vi "main_vi.vi"() -> ()   [LabVIEW 2015]
uses:
  <vilib>/Enthought/Python Integration Toolkit/api/Console Visibility.ctl
  <vilib>/Enthought/Python Integration Toolkit/api/Unpack Double.vi
  <vilib>/Enthought/Python Integration Toolkit/Python Integration Toolkit.lvlib
panel:
  out "State":string
  out "Value":dbl
  in  "Console Visibility":T1=enum."Hide Console"
  in  "Path to Python Module (.py File)":path=path ""
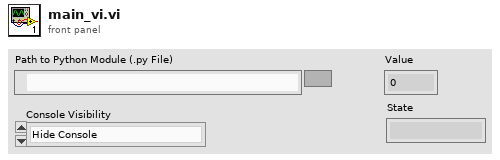
[diagram p1: front panel]
types:
  T1 = typedef "Python Integration Toolkit.lvlib/Console Visibility.ctl" = enum16{"Show Console", "Show Console While Running", "Hide Console"}
  T2 = typedef "Python Integration Toolkit.lvlib/Session ID.ctl" = u64
  T3 = typedef "Python Integration Toolkit.lvlib/Python Objects.ctl" = variant
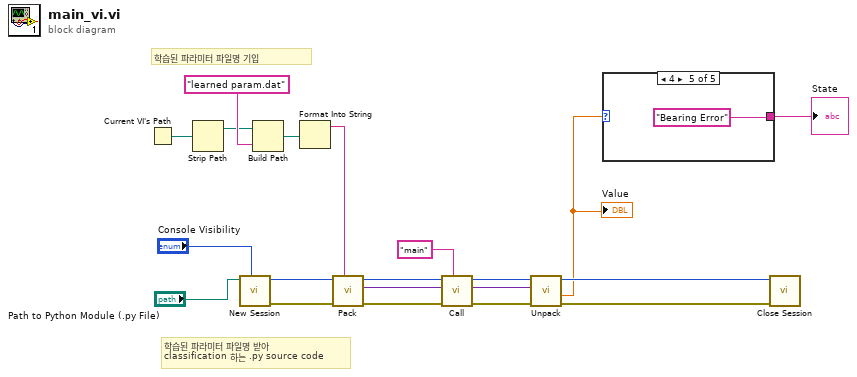
[diagram p0: block diagram]
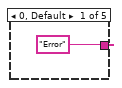
[diagram p2: hidden frame]
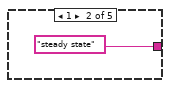
[diagram p3: hidden frame]
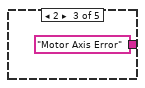
[diagram p4: hidden frame]
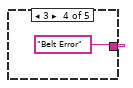
[diagram p5: hidden frame]
diagram:
  # "학습된 파라미터 파일명 받아 \nclassification 하는 .py source code"
  # "학습된 파라미터 파일명 기입"
  n1 = Current VI's Path() -> (path=w14:path)
  n2 = Strip Path(path=w14) -> (stripped path=w12:path)  [unwired: 1 out]
  n3 = call <vilib>:"New Session.vi"("Console Visibility"="Console Visibility", "Path to Python Module (.py File)"="Path to Python Module (.py File)") -> ("error out"=w9:errorcluster, "Session ID out"=w10:T2)  [unwired: 8 in]
  n4 = Build Path(base path=w12, name or relative path="learned param.dat" ("pickle path")) -> (appended path=w11:path)
  n5 = Format Into String(w11) -> (resulting string=w6:string)  [unwired: 3 in, 1 out]
  n6 = call <vilib>:"Pack.vi"("Argument"=w6, "error in (no error)"=w9, "Session ID"=w10) -> ("error out"=w7:errorcluster, "Python Object References Out"=w5:T3, "Session ID out"=w8:T2)  [unwired: 6 in]
  n7 = call <vilib>:"Call.vi"("Function or Method Name"="main", "error in (no error)"=w7, "Python Object References In"=w5, "Session ID"=w8) -> ("error out"=w19:errorcluster, "Python Object References Out"=w17:T3, "Session ID out"=w20:T2)  [unwired: 5 in]
  n8 = call-poly <vilib>:"Unpack.vi"("error in (no error)"=w19, "Python Object References In"=w17, "Session ID"=w20) -> ("error out"=w3:errorcluster, "Value"=w2:dbl, "Session ID out"=w4:T2)  [unwired: 5 in, 1 out]
  "Value" <- w2
  n9 = case shown="4" w2 {
    tunnel: ["Error" "steady state" "Motor Axis Error" "Belt Error" "Bearing Error"] -> w1
    frame 0, Default {
    }
    frame 1 {
    }
    frame 2 {
    }
    frame 3 {
    }
    frame 4 {
    }
  }
  "State" <- w1
  n10 = call <vilib>:"Close Session.vi"("error in (no error)"=w3, "Session ID"=w4) -> ()  [unwired: 9 in, 1 out]
